vi "RT Loop - Acquisition and Logging.vi"(8 "error in (no error)":errorcluster, 9 "Acquisition and Logging Configuration":T1={"Samples per Read"=1, "Number of Channels"=0, "Channel Scale Array"=[0.0, 0.0, 0.0, 0.0], "Channel Names"=[], "Trigger - RMS Value"=0.0, "Trigger - Channel"=4, "Trigger - Time (Minute)"=0, "Data Rate"=0, "# Samples After Trigger"=0}, 10 "Acquisition and Logging Queue":refnum<queue>, 11 "Message Queue":refnum<queue>) -> ()   [LabVIEW 2014]
uses:
  support/Message Queue/Message Cluster.ctl
  controls/Acquisition and Logging Configuration.ctl
  controls/FPGA VI Reference.ctl
  <vilib>/Platform/TimedLoop/XDataNode/timing_clust.ctl
  <vilib>/Platform/TimedLoop/XDataNode/nitl_modes.ctl
  <vilib>/Platform/TimedLoop/XDataNode/wakeup.ctl
  Globals/Global - Monitoring Variables.vi
  <vilib>/rvi/errors/niLvFpgaAdjustHostInterfaceError.vi
  Globals/Global - Configuration Options.vi
  <vilib>/platform/TimedLoop/XDataNode/XDataNode.xnode
  <vilib>/rvi/interface/nirviMethod/nirviMethod.xnode
  <vilib>/rvi/interface/nirviReadWriteControl/nirviReadWriteControl.xnode
  support/Message Queue/Message Queue.lvlib
  <vilib>/FPGAPlugInAG/Dynamic/niLvFpga_ReadFifo_Dynamic.vi
  <vilib>/rvi/errors/niLvFpgaMergeErrorWithErrorCode.vi
  <vilib>/Platform/TimedLoop/XDataNode/XDNodeRunTimeDep.lvlib
  NiFpgaLv.dll
  <vilib>/rvi/interface/Simulation/niFpgaSimulationCallBeginRW.vi
  <vilib>/FPGAPlugInAG/Dynamic/niLvFpga_StopFifo_Dynamic.vi
panel:
  out "Elements to be read":u32
  out "Position":u32
  out "error out":errorcluster
  in  "stop":bool
  out "Finished Late?":bool
  out "Iteration Duration":i64
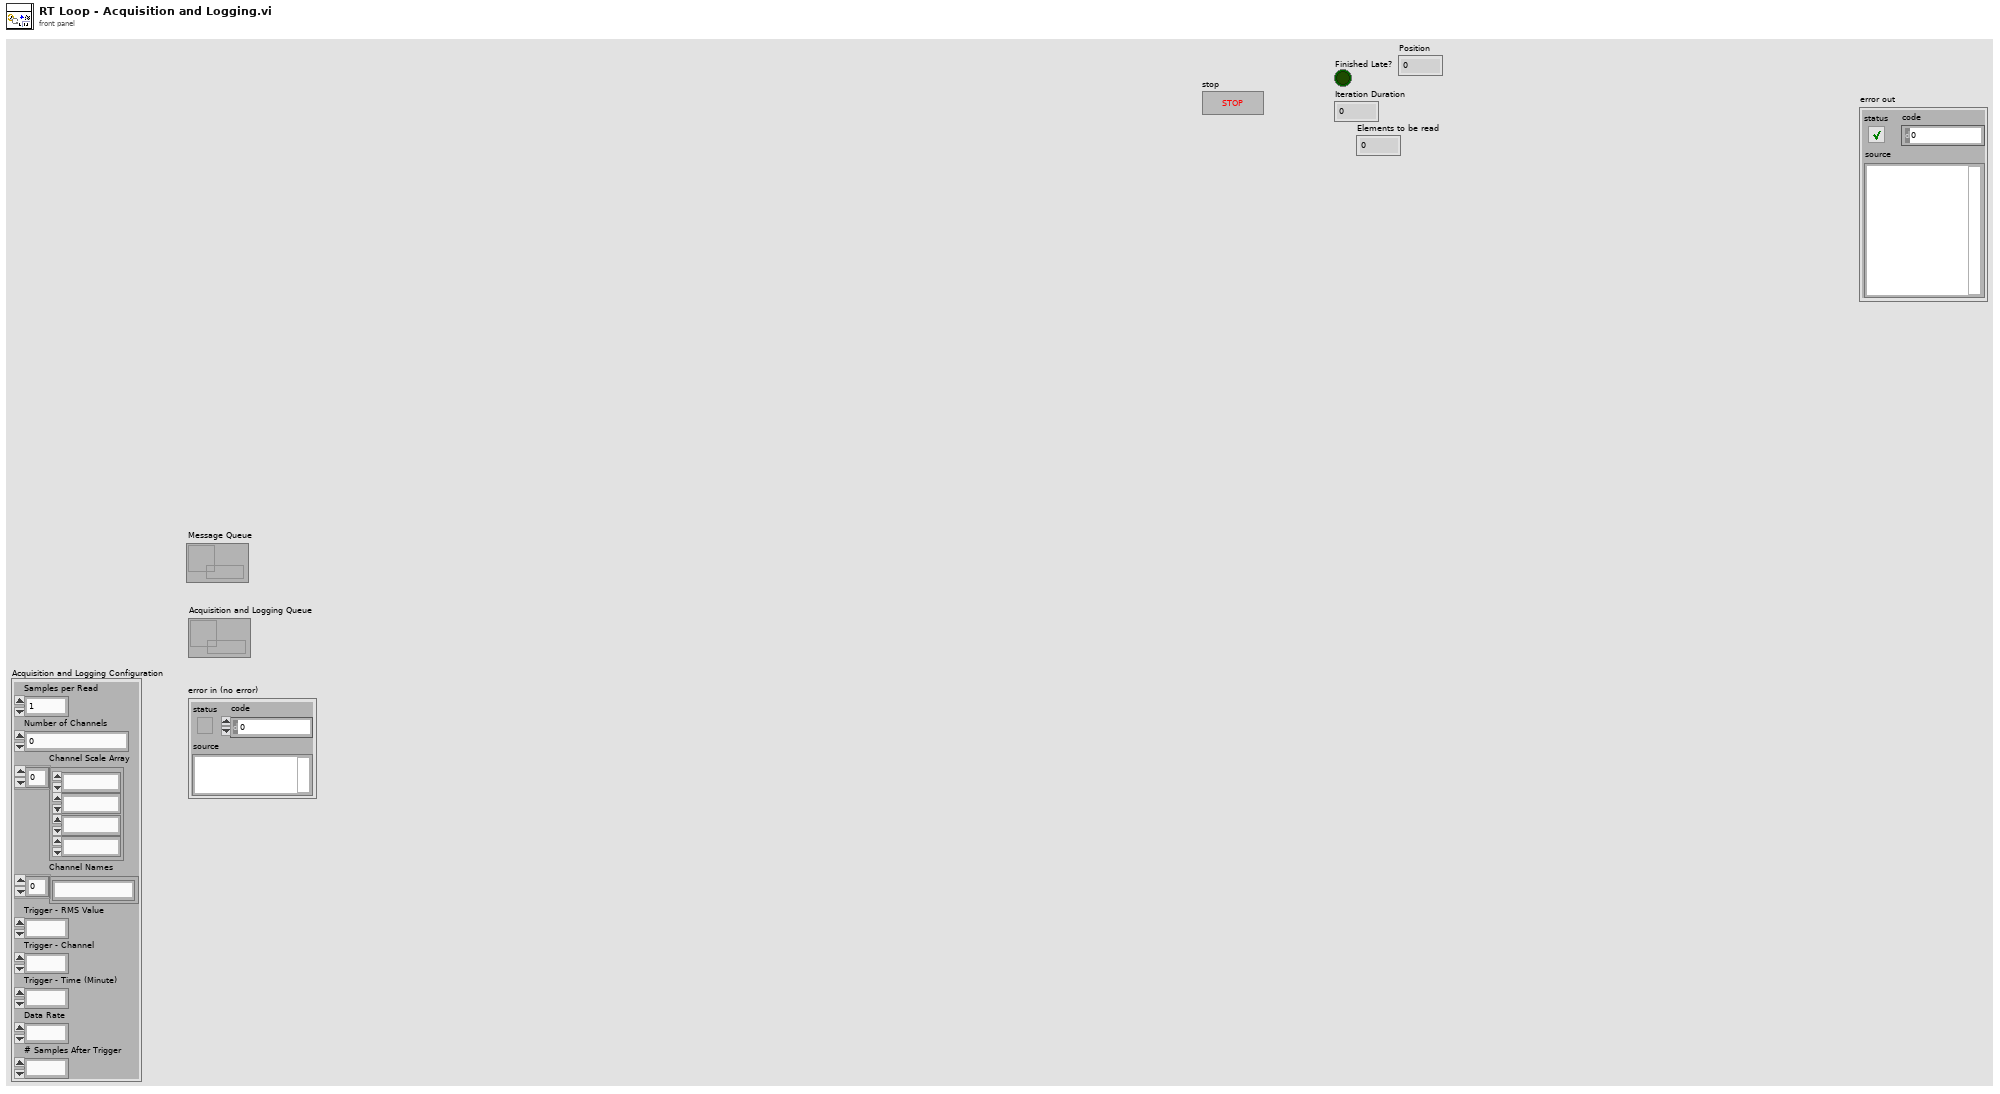
[diagram p1: front panel]
types:
  T1 = typedef "Acquisition and Logging Configuration.ctl" = cluster{"Samples per Read":i32, "Number of Channels":u32, "Channel Scale Array":fxp<+,24,12>[], "Channel Names":string[], "Trigger - RMS Value":dbl, "Trigger - Channel":i32, "Trigger - Time (Minute)":i32, "Data Rate":i32, "# Samples After Trigger":i32}
  T2 = typedef "FPGA VI Reference.ctl" = refnum<k20>
  T3 = typedef "XDNodeRunTimeDep.lvlib/timing_clust.ctl" = cluster{"Expected End [f-1]":u64, "Actual End [f-1]":u64, "Finished Late? [f-1]":bool, "Expected End [i-1]":u64, "Actual End [i-1]":u64, "Finished Late? [i-1]":bool, "Expected Start [i]":u64, "Actual Start [i]":u64, "Expected Start [f]":u64, "Actual Start [f]":u64, "Source Name":string, "Structure Name":string, "Period":i64, "Deadline":i64, "Offset":i64, "Start":i64, "Priority":i32, "Timeout":i32, "Mode":T4, "Wakeup Reason":T5, "Error":errorcluster, "Source Type":string, "Secondary Source Type":string, "Global End Time":u64, "Global Start Time":u64, "Frame Duration":u64, "Iteration Duration":u64, "Assigned CPU":i32, "I/O Scan Engine Mode":u32}
  T4 = typedef "XDNodeRunTimeDep.lvlib/nitl_modes.ctl" = enum32{"No Change", "Process missed periods, maintain original phase", "Discard missed periods, maintain original phase", "Process missed periods, ignore original phase", "Discard missed periods, ignore original phase"}
  T5 = typedef "XDNodeRunTimeDep.lvlib/wakeup.ctl" = enum32{"Normal", "Aborted", "Asynchronous wakeup", "Timing source error", "Timed loop error", "Timeout"}
  T6 = cluster{"Samples per Read":i32, "Number of Channels":u32, "Channel Scale Array":fxp<+,24,12>[], "Channel Names":string[], "Trigger - RMS Value":dbl, "Trigger - Channel":i32, "Trigger - Time (Minute)":i32, "Data Rate":i32, "# Samples After Trigger":i32}
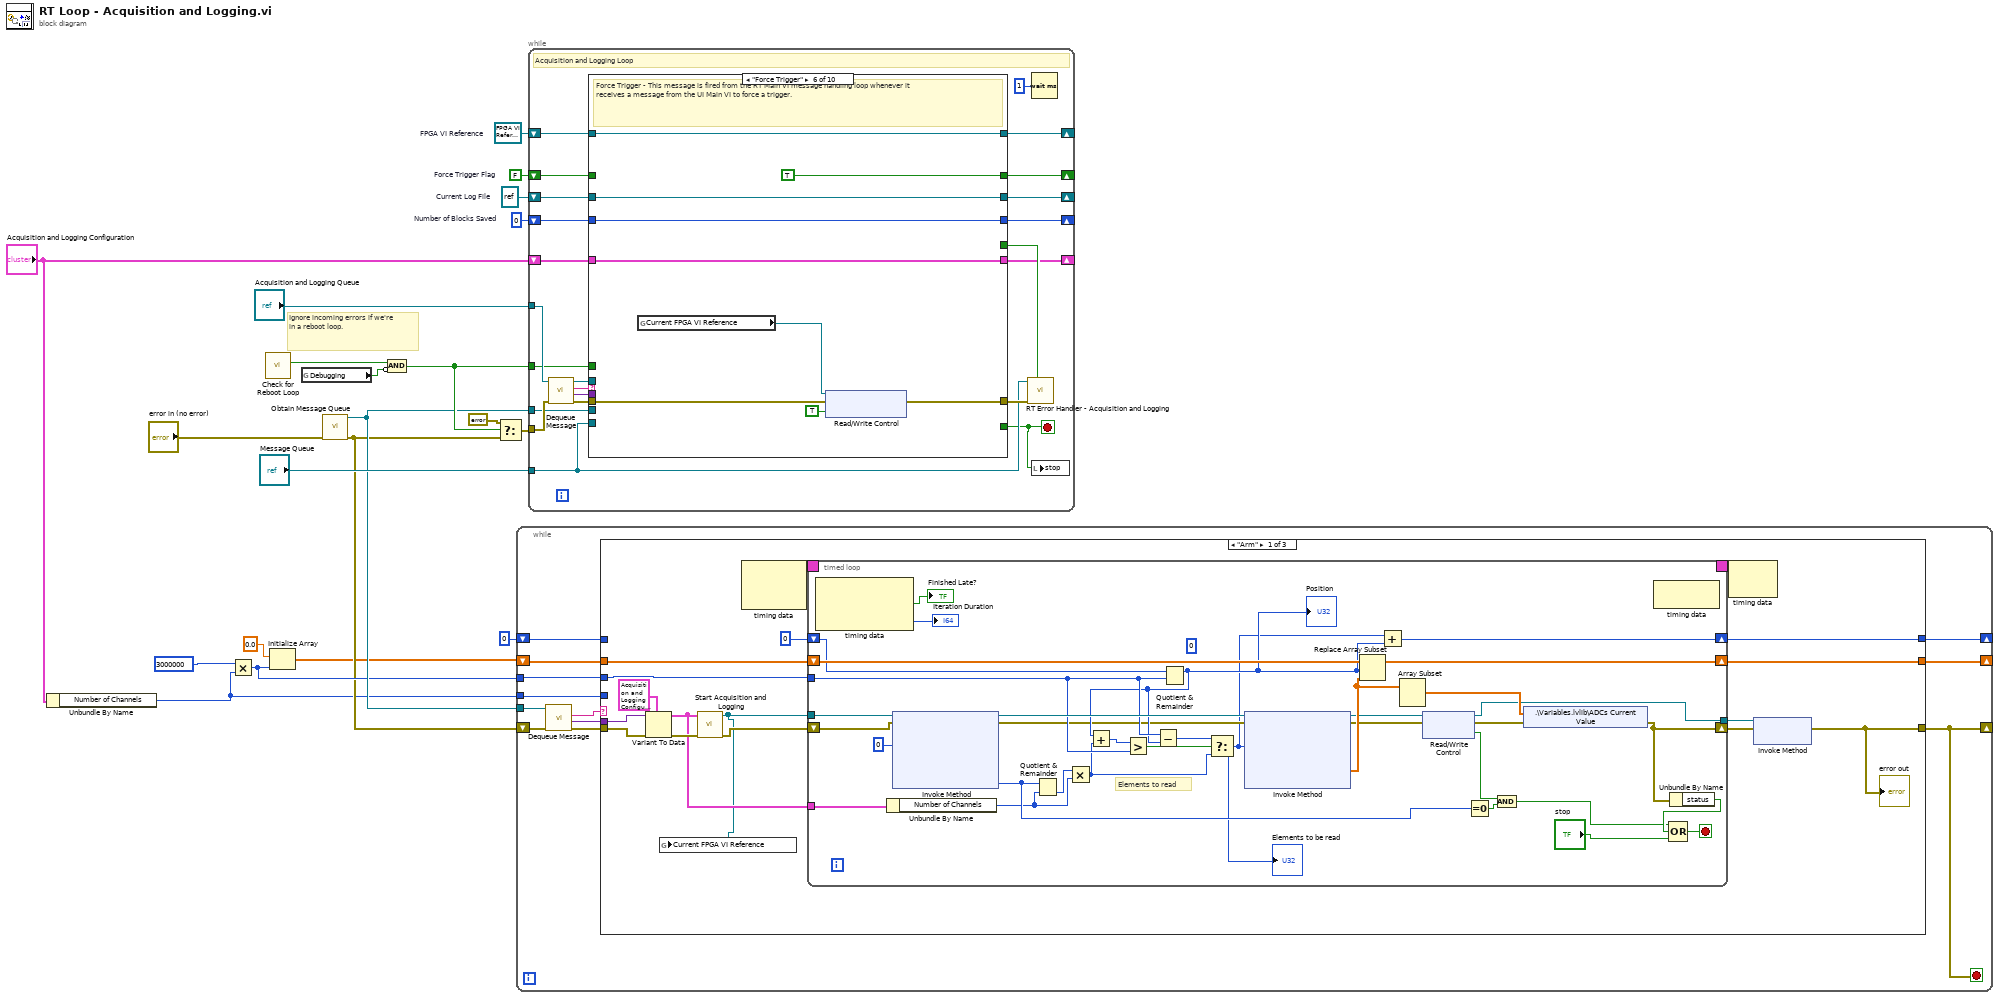
[diagram p0: block diagram]
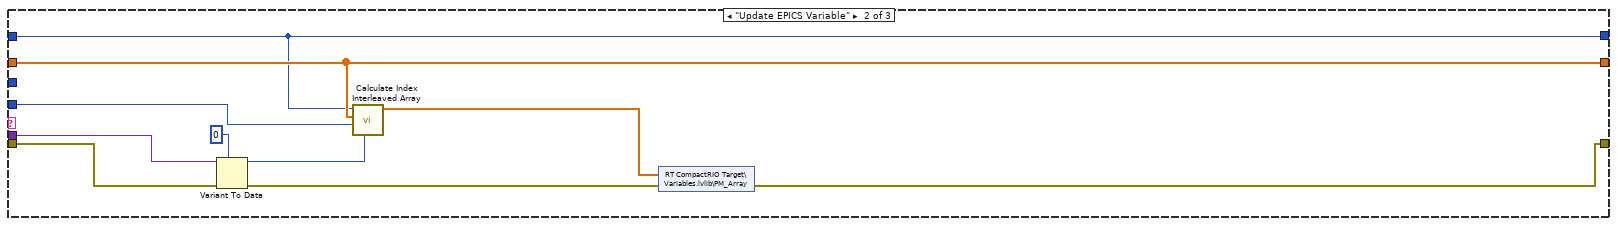
[diagram p2: hidden frame]
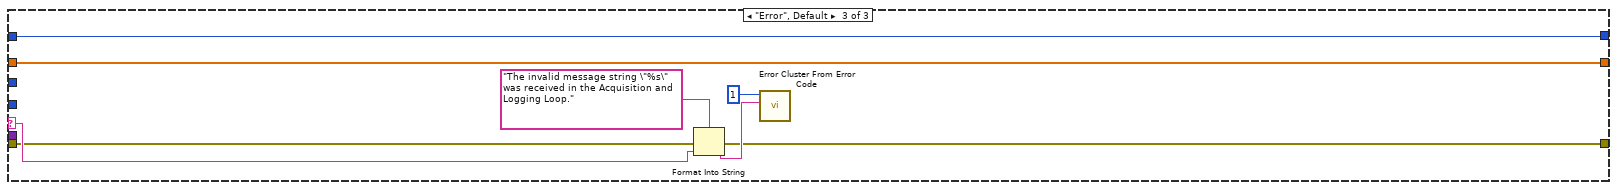
[diagram p3: hidden frame]
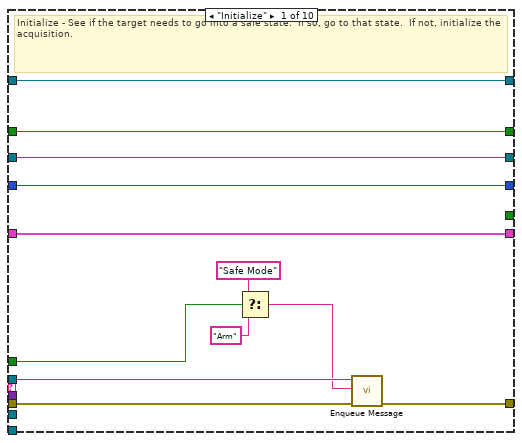
[diagram p4: hidden frame]
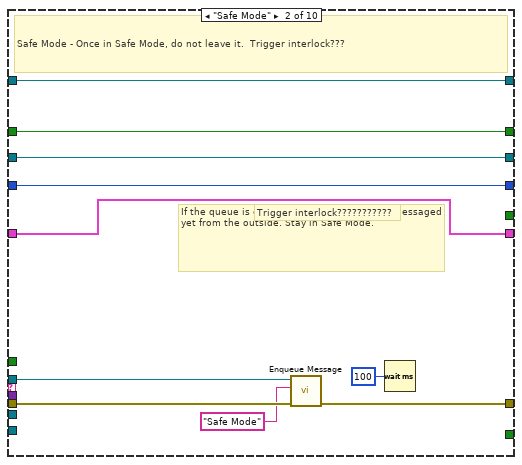
[diagram p5: hidden frame]
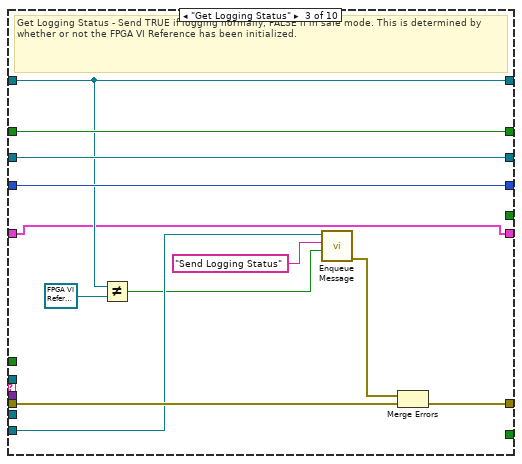
[diagram p6: hidden frame]
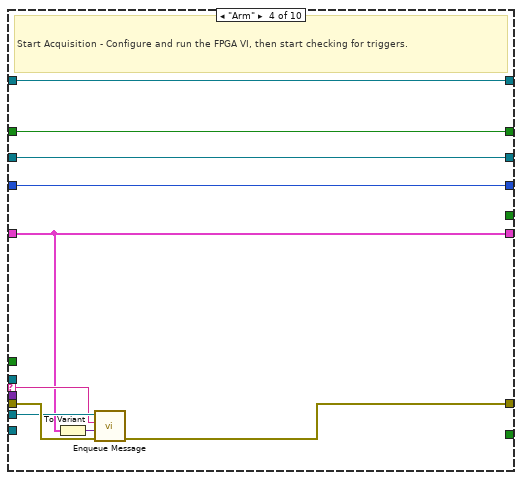
[diagram p7: hidden frame]
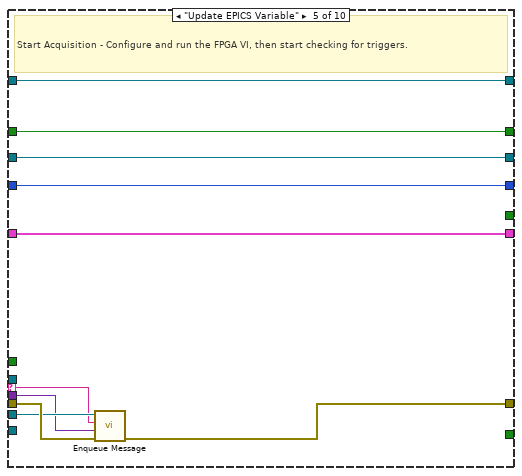
[diagram p8: hidden frame]
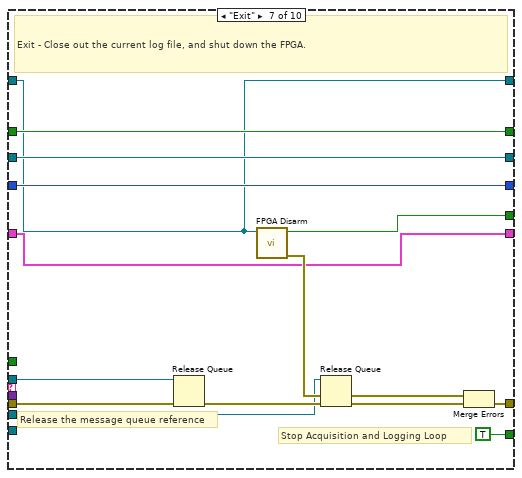
[diagram p9: hidden frame]
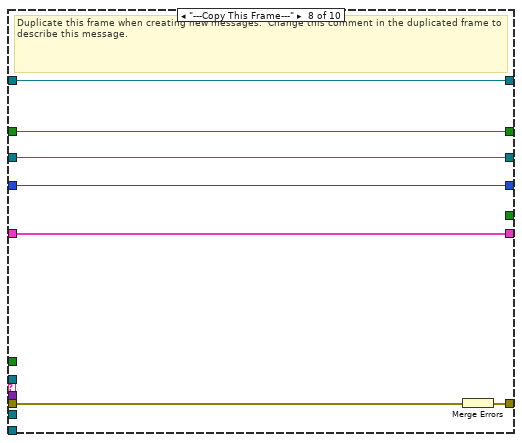
[diagram p10: hidden frame]
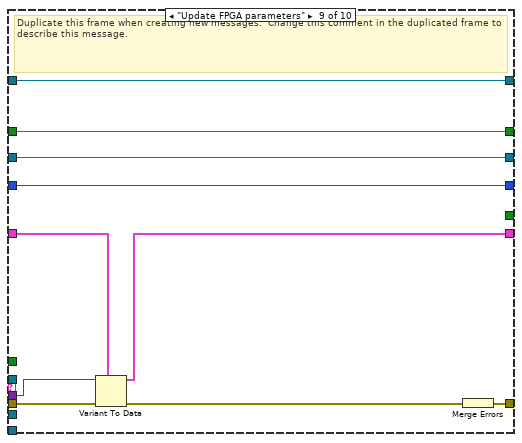
[diagram p11: hidden frame]
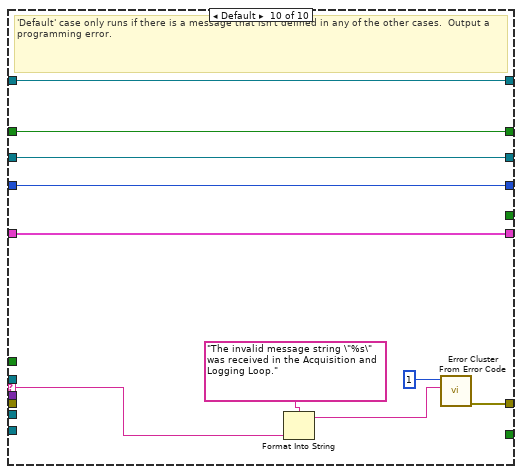
[diagram p12: hidden frame]
diagram:
  w16 = 0  # Number of Blocks Saved
  w17 = refnum<k34> refnum  # Current Log File
  w18 = FALSE  # Force Trigger Flag
  w19 = T2 refnum  # FPGA VI Reference
  # "Ignore incoming errors if we're in a reboot loop."
  n1 = Unbundle By Name("Acquisition and Logging Configuration") -> ("Number of Channels"=w1:u32)
  n2 = Multiply(x=u32 3000000 ("y"), y=w1) -> (x*y=w6:u32)
  n3 = call "Check for Reboot Loop.vi"() -> ("Start in Safe Mode?"=w13:bool)  [unwired: 10 in, 1 out]
  n4 = Initialize Array(sgl 0.0, w6) -> (w3:sgl[])
  n5 = global read "Global - Configuration Options.vi" "Debugging"() -> (w12:bool)
  n6 = call "Obtain Message Queue.vi"("error in (no error)"="error in (no error)") -> ("error out"=w4:errorcluster, "Message Queue"=w9:refnum<queue>)  [unwired: 9 in]
  n7 = Compound Arithmetic op=AND(w13, invert w12) -> (w11:bool)
  n8 = Select(t=errorcluster {"status"=FALSE, "code"=0, "source"=""}, s=w11, f=w4) -> (s? t:f=w15:errorcluster)
  n9 = while {
    tunnel: w9 -> [w28]
    shift-right: [w31] -> _
    shift-left: w4 -> [w33]
    tunnel: w6 -> [w32]
    shift-right: [w29] -> _
    shift-left: w3 -> [w30]
    shift-right: [w24] -> _
    shift-left: u32 0 ("y") -> [w23]
    tunnel: w1 -> [w22]
    stop <- w31 stop-if-true
    n10 = call "Dequeue Message.vi"("error in (no error)"=w33, "Message Queue"=w28) -> ("error out"=w25:errorcluster, "Message Data"=w26:variant, "Message"=w27:string)  [unwired: 6 in, 1 out]
    n11 = case shown="\"Arm\"" w27 {
      selector: w27 -> [_ _ w105]
      tunnel: [w36 w92 w103] -> w31
      tunnel: w32 -> [w46 _ _]
      tunnel: w30 -> [w45 w97 w109]
      tunnel: [w44 w97 w109] -> w29
      tunnel: w26 -> [w43 w101 _]
      tunnel: w25 -> [w42 w100 w104]
      tunnel: [w39 w96 w102] -> w24
      tunnel: w23 -> [_ w96 w102]
      tunnel: w22 -> [_ w95 _]
      frame "Arm" {
        n12 = Variant To Data(error in=w42, type=T1 {"Samples per Read"=0, "Number of Channels"=16, "Channel Scale Array"=[0.0, 0.0, 0.0, 0.0], "Channel Names"=[], "Trigger - RMS Value"=0.0, "Trigger - Channel"=0, "Trigger - Time (Minute)"=0, "Data Rate"=100000, "# Samples After Trigger"=0} ("Acquisition and Logging Configuration"), Variant=w43) -> (data=w38:T6, error out=w41:errorcluster)
        n13 = call "Start Acquisition and Logging.vi"("error in (no error)"=w41, "Acquisition and Logging Configuration"=w38) -> ("error out"=w48:errorcluster, "FPGA VI Reference"=w34:T2)  [unwired: 7 in, 1 out]
        n14 = global write "Global - Monitoring Variables.vi" "Current FPGA VI Reference"(w34) -> ()
        n15 = node-c288() -> (w50:T3)  [unwired: 2 in]
        n16 = timed-loop {
          tunnel: w34 -> [w75]
          shift-right: [w83] -> w44
          shift-left: w45 -> [w84]
          tunnel: w46 -> [w63]
          timing: w50 -> [_]
          timing-out: [_] -> w49
          shift-right: [w55] -> w39
          shift-left: u32 0 ("y") -> [w60]
          shift-right: [w69] -> w37
          shift-left: w48 -> [w76]
          tunnel: w38 -> [w53]
          tunnel: [w51] -> w35
          stop <- w57 stop-if-true
          (unwired) u32 0
          # "Elements to read"
          n17 = node-c288() -> (→"Finished Late?":bool, →"Iteration Duration":i64)  [unwired: 1 in, 1 out]
          n18 = Unbundle By Name(w53) -> ("Number of Channels"=w52:u32)
          n19 = xnode "Invoke Method"("FPGA VI Reference In"=w75, "error in"=w76, "Number of Elements"=u32 0) -> ("FPGA VI Reference Out"=w74:T2, "error out"=w56:errorcluster, "Elements Remaining"=w65:u32)  [unwired: 1 in, 1 out]
          n20 = Quotient & Remainder(x=w65, y=w52) -> (floor(x/y)=w73:u32)  [unwired: 1 out]
          n21 = Multiply(x=w73, y=w52) -> (x*y=w58:u32)
          n22 = Quotient & Remainder(x=w60, y=w63) -> (x-y*floor(x/y)=w62:u32)  [unwired: 1 out]
          "Position" <- w62
          n23 = Add(x=w62, y=w58) -> (x+y=w59:u32)
          n24 = Greater?(x=w59, y=w63) -> (0:w64:bool)
          n25 = Subtract(x=w63, y=w62) -> (x-y=w61:u32)
          n26 = Select(t=w61, s=w64, f=w58) -> (s? t:f=w54:u32)
          "Elements to be read" <- w54
          n27 = xnode "Invoke Method"("FPGA VI Reference In"=w74, "error in"=w56, "Number of Elements"=w54) -> ("FPGA VI Reference Out"=w72:T2, "error out"=w71:errorcluster, "Data"=w82:sgl[])  [unwired: 1 in, 1 out]
          n28 = Replace Array Subset(array=w84, new element=w82, index=w62) -> (w83:sgl[])
          n29 = Add(x=w54, y=w62) -> (x+y=w55:u32)
          n30 = Array Subset(array=w82) -> (w85:sgl[])  [unwired: 2 in]
          n31 = xnode "Read/Write Control"("FPGA VI Reference In"=w72, "error in"=w71) -> ("FPGA VI Reference Out"=w51:T2, "error out"=w70:errorcluster, "Stopped"=w68:bool)
          n32 = Equal To 0?(x=w65) -> (x = 0?=w66:bool)
          n33 = And(x=w68, y=w66) -> (x .and. y?=w67:bool)
          n34 = shared-variable ".\\Variables.lvlib\\ADCs Current Value"(w85, error in=w70) -> (error out=w69:errorcluster)
          n35 = node-c288() -> ()  [unwired: 1 in, 1 out]
          n36 = Unbundle By Name(w69) -> ("status"=w81:bool)
          n37 = Compound Arithmetic op=OR(w67, w81, "stop") -> (w57:bool)
        }
        n38 = node-c288(w49) -> ()  [unwired: 1 out]
        n39 = xnode "Invoke Method"("FPGA VI Reference In"=w35, "error in"=w37) -> ("error out"=w36:errorcluster)  [unwired: 1 out]
        "error out" <- w36
      }
      frame "Update EPICS Variable" {
        n40 = Variant To Data(error in=w100, type=0, Variant=w101) -> (data=w98:i32, error out=w93:errorcluster)
        n41 = call "Calculate Index Interleaved Array.vi"("Index"=w98, "Number of Channels"=w95, "Interleaved Array"=w97, "Position Zero"=w96) -> ("Array"=w94:sgl[])  [unwired: 7 in]
        n42 = shared-variable "RT CompactRIO Target\\Variables.lvlib\\PM_Array"(w94, error in=w93) -> (error out=w92:errorcluster)
      }
      frame "Error", Default {
        n43 = Format Into String(format string="The invalid message string \"%s\" was received in the Acquisition and Logging Loop." ("Unknown Message Error Text"), error in=w104, w105) -> (resulting string=w106:string, error out=w103:errorcluster)  [unwired: 1 in]
        n44 = call <vilib>:"Error Cluster From Error Code.vi"("error message (\"\")"=w106, "error code (0)"=1) -> ()  [unwired: 7 in, 1 out]
      }
    }
  }
  n45 = while {
    tunnel: "Acquisition and Logging Queue" -> [w129]
    tunnel: "Message Queue" -> [w116]
    shift-right: [w125] -> _
    shift-left: w19 -> [w126]
    shift-right: [w121] -> _
    shift-left: w18 -> [w122]
    shift-right: [w119] -> _
    shift-left: w17 -> [w120]
    shift-right: [w117] -> _
    shift-left: w16 -> [w118]
    tunnel: w15 -> [w114]
    tunnel: w11 -> [w113]
    tunnel: w9 -> [w111]
    shift-right: [w110] -> _
    shift-left: "Acquisition and Logging Configuration" -> [w124]
    stop <- w112 stop-if-true
    # "Acquisition and Logging Loop"
    n46 = call "Dequeue Message.vi"("error in (no error)"=w114, "Message Queue"=w129) -> ("error out"=w132:errorcluster, "Message Data"=w130:variant, "Message"=w131:string, "dup Message Queue"=w127:refnum<queue>)  [unwired: 6 in]
    n47 = case "Message Cases" shown="\"Force Trigger\"" w131 {
      selector: w131 -> [_ _ _ w169 w179 _ _ _ _ w235]
      tunnel: w127 -> [w142 w152 _ _ _ _ w209 _ _ _]
      tunnel: w132 -> [w143 w153 w166 w173 w183 w190 w205 w216 w219 _]
      tunnel: [w135 w151 w160 w172 w182 w189 w206 w215 w226 w233] -> w128
      tunnel: [_ _ _ _ _ _ TRUE _ _ _] -> w112
      tunnel: w130 -> [_ _ _ _ w178 _ _ _ w221 _]
      tunnel: w126 -> [w144 w154 w162 w171 w181 w195 w199 w214 w225 w231]
      tunnel: [w144 w154 w162 w171 w181 w195 w199 w214 w225 w231] -> w125
      tunnel: w124 -> [w133 w145 w155 w167 w177 w191 w198 w210 w220 w227]
      tunnel: w122 -> [w138 w150 w165 w176 w186 _ w203 w213 w224 w230]
      tunnel: [w138 w150 w165 w176 w186 TRUE ("Force Trigger Flag") w203 w213 w224 w230] -> w121
      tunnel: w120 -> [w137 w149 w164 w175 w185 w194 w201 w212 w223 w229]
      tunnel: [w137 w149 w164 w175 w185 w194 w201 w212 w223 w229] -> w119
      tunnel: w118 -> [w136 w148 w163 w174 w184 w192 w202 w211 w222 w228]
      tunnel: [w136 w148 w163 w174 w184 w192 w202 w211 w222 w228] -> w117
      tunnel: w116 -> [_ _ w161 _ _ _ _ _ _ _]
      tunnel: [_ _ _ _ _ _ w200 _ _ _] -> w115
      tunnel: w113 -> [w134 _ _ _ _ _ _ _ _ _]
      tunnel: w111 -> [_ _ _ w170 w180 _ w196 _ _ _]
      tunnel: [w133 w145 w155 w167 w177 w191 w198 w210 w217 w227] -> w110
      frame "Initialize" {
        # "Initialize - See if the target needs to go into a safe state.  If so, go to that state.  If not, initialize the acquisition."
        n48 = Select(t="Safe Mode", s=w134, f="Arm") -> (s? t:f=w139:string)
        n49 = call "Enqueue Message.vi"("error in (no error)"=w143, "Message"=w139, "Message Queue"=w142) -> ("error out"=w135:errorcluster)  [unwired: 7 in, 1 out]
      }
      frame "Safe Mode" {
        # "Trigger interlock???????????"
        # "If the queue is empty, this loop hasn't been messaged yet from the outside. Stay in Safe Mode."
        # "Safe Mode - Once in Safe Mode, do not leave it.  Trigger interlock???"
        n50 = call "Enqueue Message.vi"("error in (no error)"=w153, "Message"="Safe Mode", "Message Queue"=w152) -> ("error out"=w151:errorcluster)  [unwired: 7 in, 1 out]
        n51 = Wait (ms)(milliseconds to wait=u32 100) -> ()  [unwired: 1 out]
      }
      frame "Get Logging Status" {
        # "Get Logging Status - Send TRUE if logging normally, FALSE if in safe mode. This is determined by whether or not the FPGA VI Reference has been initialized."
        n52 = Not Equal?(x=w162, y=T2 refnum ("FPGA VI Reference")) -> (x != y?=w158:bool)
        n53 = call "Enqueue Message.vi"("Message Data"=w158, "Message"="Send Logging Status", "Message Queue"=w161) -> ("error out"=w159:errorcluster)  [unwired: 7 in, 1 out]
        n54 = Merge Errors(w159, w166) -> (w160:errorcluster)
      }
      frame "Arm" {
        # "Start Acquisition - Configure and run the FPGA VI, then start checking for triggers."
        n55 = To Variant(anything=w167) -> (Variant=w168:variant)
        n56 = call "Enqueue Message.vi"("error in (no error)"=w173, "Message Data"=w168, "Message"=w169, "Message Queue"=w170) -> ("error out"=w172:errorcluster)  [unwired: 6 in, 1 out]
      }
      frame "Update EPICS Variable" {
        # "Start Acquisition - Configure and run the FPGA VI, then start checking for triggers."
        n57 = call "Enqueue Message.vi"("error in (no error)"=w183, "Message Data"=w178, "Message"=w179, "Message Queue"=w180) -> ("error out"=w182:errorcluster)  [unwired: 6 in, 1 out]
      }
      frame "Force Trigger" {
        # "Force Trigger - This message is fired from the RT Main VI message handling loop whenever it receives a message from the UI Main VI to force a trigger."
        n58 = global read "Global - Monitoring Variables.vi" "Current FPGA VI Reference"() -> (w188:T2)
        n59 = xnode "Read/Write Control"("FPGA VI Reference In"=w188, "error in"=w190, "External trigger"=TRUE) -> ("error out"=w189:errorcluster)  [unwired: 1 out]
      }
      frame "Exit" {
        # "Stop Acquisition and Logging Loop"
        # "Release the message queue reference"
        # "Exit - Close out the current log file, and shut down the FPGA."
        n60 = Release Queue(queue=w209, error in (no error)=w205) -> (error out=w207:errorcluster)  [unwired: 1 in, 2 out]
        n61 = call "FPGA Disarm.vi"("FPGA VI Reference"=w199) -> ("error out"=w204:errorcluster, "Stop FPGA Timeout?"=w200:bool)  [unwired: 9 in]
        n62 = Release Queue(queue=w196, error in (no error)=w207) -> (error out=w197:errorcluster)  [unwired: 1 in, 2 out]
        n63 = Merge Errors(w204, w197) -> (w206:errorcluster)
      }
      frame "---Copy This Frame---" {
        # "Duplicate this frame when creating new messages.  Change this comment in the duplicated frame to describe this message."
        n64 = Merge Errors(w216) -> (w215:errorcluster)
      }
      frame "Update FPGA parameters" {
        # "Duplicate this frame when creating new messages.  Change this comment in the duplicated frame to describe this message."
        n65 = Variant To Data(error in=w219, type=w220, Variant=w221) -> (data=w217:T6, error out=w218:errorcluster)
        n66 = Merge Errors(w218) -> (w226:errorcluster)
      }
      frame Default {
        # "'Default' case only runs if there is a message that isn't defined in any of the other cases.  Output a programming error."
        n67 = Format Into String(format string="The invalid message string \"%s\" was received in the Acquisition and Logging Loop." ("Unknown Message Error Text"), w235) -> (resulting string=w232:string)  [unwired: 2 in, 1 out]
        n68 = call <vilib>:"Error Cluster From Error Code.vi"("error message (\"\")"=w232, "error code (0)"=1) -> ("error out"=w233:errorcluster)  [unwired: 7 in]
      }
    }
    n69 = call "RT Error Handler - Acquisition and Logging.vi"("Stop FPGA Timeout"=w115, "error in (no error)"=w128, "Message Queue"=w116) -> ()  [unwired: 8 in, 1 out]
    n70 = local write "stop"(w112) -> ()
    n71 = Wait (ms)(milliseconds to wait=u32 1) -> ()  [unwired: 1 out]
  }
